vi "DrawCross.vi"(9 "Rotation":dbl format="%#_13g", 10 "Position":cluster{"x":sgl, "y":sgl}, 11 "Image":T1) -> (3 "Image Out":T1)   [LabVIEW 2014]
uses:
  <vilib>/vision/Image Controls.llb/IMAQ Image.ctl
  <vilib>/Analysis/coordinate.llb/2D Cartesian Coordinate Rotation (Scalar).vi
  <vilib>/Analysis/NI_AALPro.lvlib
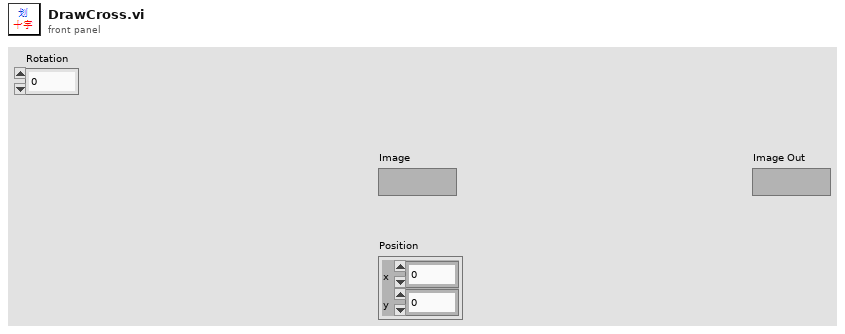
[diagram p1: front panel]
types:
  T1 = typedef "IMAQ Image.ctl" = refnum<image>
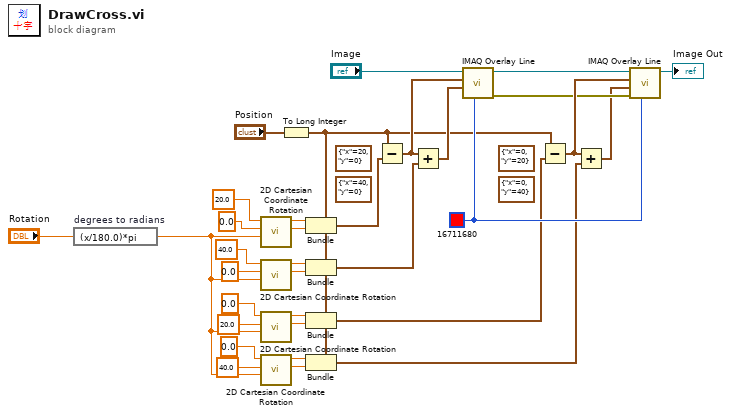
[diagram p0: block diagram]
diagram:
  w26 = u32 16711680 ("Color")
  (unwired) cluster{"x":i32, "y":i32} {"x"=0, "y"=40} ("y")
  (unwired) cluster{"x":i32, "y":i32} {"x"=0, "y"=20} ("y")
  (unwired) cluster{"x":i32, "y":i32} {"x"=40, "y"=0} ("y")
  (unwired) cluster{"x":i32, "y":i32} {"x"=20, "y"=0} ("y")
  n1 = expression code="(x/180.0)*pi" "degrees to radians"("Rotation") -> (w22:dbl)
  n2 = call-poly <vilib>:"2D Cartesian Coordinate Rotation.vi"("theta"=w22, "y"=0.0 ("Numeric"), "x"=20.0 ("Numeric")) -> ("y out"=w12:dbl, "x out"=w13:dbl)  [unwired: 6 in, 1 out]
  n3 = call-poly <vilib>:"2D Cartesian Coordinate Rotation.vi"("theta"=w22, "y"=0.0 ("Numeric"), "x"=40.0 ("Numeric")) -> ("y out"=w10:dbl, "x out"=w11:dbl)  [unwired: 6 in, 1 out]
  n4 = call-poly <vilib>:"2D Cartesian Coordinate Rotation.vi"("theta"=w22, "y"=20.0 ("Numeric"), "x"=0.0 ("Numeric")) -> ("y out"=w8:dbl, "x out"=w9:dbl)  [unwired: 6 in, 1 out]
  n5 = call-poly <vilib>:"2D Cartesian Coordinate Rotation.vi"("theta"=w22, "y"=40.0 ("Numeric"), "x"=0.0 ("Numeric")) -> ("y out"=w6:dbl, "x out"=w7:dbl)  [unwired: 6 in, 1 out]
  n6 = To Long Integer(number="Position") -> (32bit integer=w5:cluster{"x":i32, "y":i32})
  n7 = Bundle(cluster=w5, "x"=w13, "y"=w12) -> (w4:cluster{"x":i32, "y":i32})
  n8 = Bundle(cluster=w5, "x"=w11, "y"=w10) -> (w3:cluster{"x":i32, "y":i32})
  n9 = Bundle(cluster=w5, "x"=w9, "y"=w8) -> (w2:cluster{"x":i32, "y":i32})
  n10 = Bundle(cluster=w5, "x"=w7, "y"=w6) -> (w1:cluster{"x":i32, "y":i32})
  n11 = Subtract(x=w5, y=w4) -> (x-y=w33:cluster{"x":i32, "y":i32})
  n12 = Add(x=w33, y=w3) -> (x+y=w32:cluster{"x":i32, "y":i32})
  n13 = call "IMAQ Overlay Line"("Color"=w26, "End Point"=w32, "Start Point"=w33, "Image"="Image") -> ("error out"=w29:errorcluster, "Image Out"=w30:T1)  [unwired: 2 in, 4 out]
  n14 = Subtract(x=w5, y=w2) -> (x-y=w31:cluster{"x":i32, "y":i32})
  n15 = Add(x=w31, y=w1) -> (x+y=w27:cluster{"x":i32, "y":i32})
  n16 = call "IMAQ Overlay Line"("Color"=w26, "error in (no error)"=w29, "End Point"=w27, "Start Point"=w31, "Image"=w30) -> ("Image Out"=→"Image Out":T1)  [unwired: 1 in, 5 out]
